vi "Virtual Axis Move at Velocity (Polymorphic).vi"   [LabVIEW 2013, in "Zaber A Series.lvlib"]
doc: "Moves a virtual axis at a specified speed. The move speed can be specified for the virtual axis itself or for one of the physical axes comprising it, in which case the other axes will move at proportional speeds.\n\nThe move speed is specified in microstep units for the axis selected. Use the Convert Velocity Units to Device Units VI to convert from standard distance units.\n\nNo responses are returned with this VI, but if you would like to wait until the movement is completed to continue, you can combine this VI with the Poll Until Idle VI. \n\nThis VI requires that the Initialize VI has been called with the same serial port and that the lockstep group has been created with the Lockstep Enable VI."
uses:
  Zaber A Series.lvlib
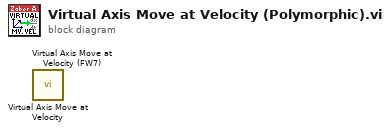
[diagram p0: block diagram]
diagram:
  n1 = call "Virtual Axis Move at Velocity.vi"() -> ()  [unwired: 10 in, 2 out]
  n2 = call "Virtual Axis Move at Velocity (FW7).vi"() -> ()  [unwired: 10 in, 2 out]
